vi "XY图（椭圆）.vi"() -> ()   [LabVIEW 2017]
panel:
  out "XY图":cluster{dbl[], dbl[]}(graph)
  in  "b":dbl(knob) scale=0.0..10.0
  in  "a":dbl(knob) scale=0.0..10.0
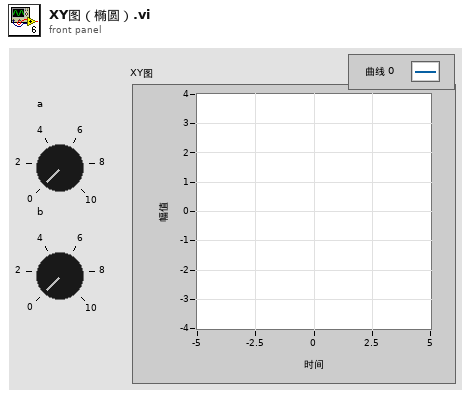
[diagram p1: front panel]
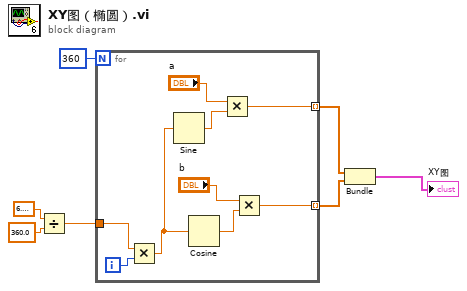
[diagram p0: block diagram]
diagram:
  n1 = Divide(x=6.283185307179586, y=360.0) -> (x/y=w5:dbl)
  n2 = for {
    N: 360 -> [_]
    tunnel: w5 -> [w15]
    tunnel: [w9] -> w4 mode=indexing
    tunnel: [w8] -> w3 mode=indexing
    i -> [w16]
    n3 = Multiply(x=w15, y=w16) -> (x*y=w14:dbl)
    n4 = Sine(x=w14) -> (sin(x)=w11:dbl)
    n5 = Cosine(x=w14) -> (cos(x)=w13:dbl)
    n6 = Multiply(x="a", y=w11) -> (x*y=w9:dbl)
    n7 = Multiply(x="b", y=w13) -> (x*y=w8:dbl)
  }
  n8 = Bundle(w4, w3) -> (→"XY图":cluster{dbl[], dbl[]})  [unwired: 1 in]
